vi "LastCoordinatesFunction.vi"(10 "YArray":dbl[](array[numeric]), 11 "XArray":dbl[](array[numeric])) -> (2 "LastYCoordinate":dbl, 3 "LastXCoordinate":dbl)   [LabVIEW 2017]
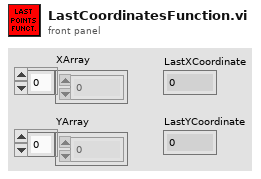
[diagram p1: front panel]
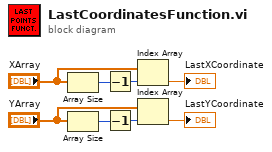
[diagram p0: block diagram]
diagram:
  n1 = Array Size(array="XArray") -> (size(s)=w8:i32)
  n2 = Array Size(array="YArray") -> (size(s)=w4:i32)
  n3 = Decrement(x=w8) -> (x-1=w7:i32)
  n4 = Decrement(x=w4) -> (x-1=w3:i32)
  n5 = Index Array(array="XArray", index=w7) -> (element=→"LastXCoordinate":dbl)
  n6 = Index Array(array="YArray", index=w3) -> (element=→"LastYCoordinate":dbl)
